vi "event_based_motor_control.vi"() -> ()   [LabVIEW 2025]
panel:
  out "Current position (units)":dbl format="%.2f"
  in  "stop":bool
  in  "New target position (units)":dbl format="%.2f"
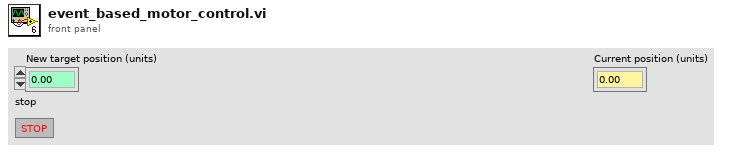
[diagram p1: front panel]
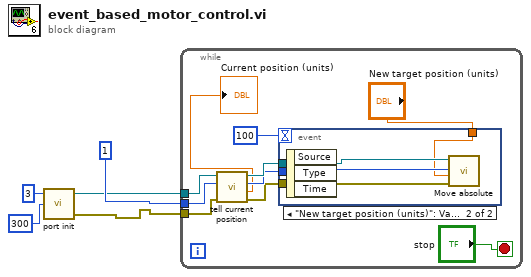
[diagram p0: block diagram]
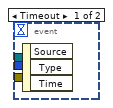
[diagram p2: hidden frame]
diagram:
  n1 = call <userlib>:"port init.vi"("Timeout (ms)"=u32 300, "SerialPort"=u8 3) -> ("error out"=w1:errorcluster, "Visa Handle"=w2:refnum<visa-resource-name>)  [unwired: 2 in]
  n2 = while {
    tunnel: w1 -> [w10]
    tunnel: w2 -> [w12]
    tunnel: 1 ("Axis in in") -> [w11]
    stop <- "stop" stop-if-true
    n3 = call <userlib>:"tell current position.vi"("error in"=w10, "Axis in"=w11, "VISA Handle in"=w12) -> ("error out"=w6:errorcluster, "Current position (units)"=→"Current position (units)":dbl, "Axis out"=w8:i32, "VISA Handle out"=w9:refnum<visa-resource-name>)  [unwired: 2 in, 1 out]
    n4 = event shown="[1] \"New target position (units)\": Value Change" {
      selector: _ -> [_ _]
      dyn-events: _ -> [_ _]
      timeout: 100 -> [_ _]
      tunnel: "New target position (units)" -> [_ w16]
      tunnel: w9 -> [_ w19]
      tunnel: w6 -> [_ w17]
      tunnel: w8 -> [_ w18]
      event Timeout {
        n5 = event-data() -> ()  [unwired: 1 in, 3 out]
      }
      event "New target position (units)": Value Change {
        n6 = event-data() -> ()  [unwired: 1 in, 3 out]
        n7 = call <userlib>:"Move absolute.vi"("error in"=w17, "New target position (units)"=w16, "Axis in"=w18, "VISA Handle in"=w19) -> ()  [unwired: 2 in, 4 out]
      }
    }
  }
